vi "Write Night Directory.vi"(8 "error in (no error)":errorcluster, 10 "Directory":string, 11 "Setup File in":refnum<class "Setup File.lvclass">) -> (0 "error out":errorcluster, 3 "Setup File out":refnum<class "Setup File.lvclass">)   [LabVIEW 2018, in "Setup File.lvclass"]
uses:
  Setup File.lvclass
  Setup File.lvclass/Setup File.ctl
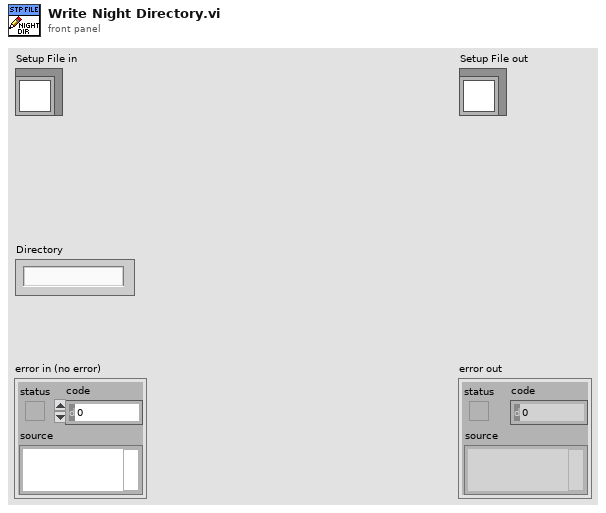
[diagram p1: front panel]
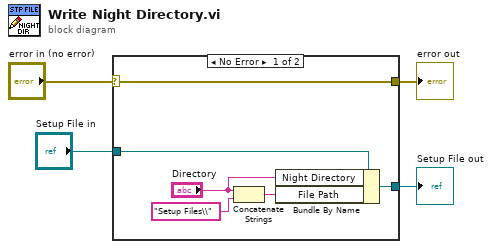
[diagram p0: block diagram]
diagram:
  n1 = case shown="No Error" "error in (no error)" {
    selector: "error in (no error)" -> [w10 w11]
    tunnel: [w10 w11] -> w2
    tunnel: [w8 w12] -> w1
    tunnel: "Setup File in" -> [w9 w12]
    frame No Error {
      n2 = Concatenate Strings("Directory", "Setup Files\\") -> (w5:string)
      n3 = Bundle By Name(cluster=w9, "Night Directory"="Directory", "File Path"=w5) -> (w8:refnum<class "Setup File.lvclass">)
    }
    frame Error {
    }
  }
  "error out" <- w2
  "Setup File out" <- w1
